vi "Set 2D Ramp Rates.vi"(0 "Y-Axis Communications Config":T1={"GPIB address"=22, "GPIB bus"=0, "connection ID"=refnum, "IP"="192.168.2.200", "Active Comm Interface"=0, "Serial Port"="", "Programmer Type"=0} {"Programmer Type" items=["Model 430", "Model 420"]; "Active Comm Interface" items=["TCP/IP (Model 430 Only)", "RS232", "IEEE488"]}, 1 "Y-Axis Field (kG)":dbl format="%.3f", 3 "Next Y-Axis Field (kG)":dbl format="%.3f", 4 "Z-Axis Communications Config":T1={"GPIB address"=22, "GPIB bus"=0, "connection ID"=refnum, "IP"="192.168.2.200", "Active Comm Interface"=0, "Serial Port"="", "Programmer Type"=0} {"Programmer Type" items=["Model 430", "Model 420"]; "Active Comm Interface" items=["TCP/IP (Model 430 Only)", "RS232", "IEEE488"]}, 5 "Z-Axis Field (kG)":dbl format="%.3f", 7 "Next Z-Axis Field (kG)":dbl format="%.3f", 8 "Max Ramp Rate - Y Axis (A/s)":dbl format="%.3f", 9 "Max Ramp Rate - Z Axis (A/s)":dbl format="%.3f", 11 "error in":T2) -> (15 "Y-Axis Ramp Rate (kG/s)":dbl format="%.3f", 17 "Z-Axis Ramp Rate (kG/s)":dbl format="%.3f", 18 "error out":T2)   [LabVIEW 2016]
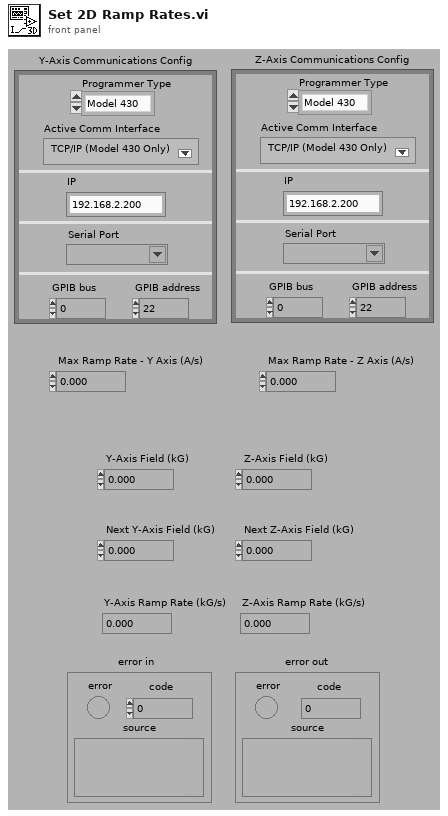
[diagram p1: front panel]
types:
  T1 = cluster{"GPIB address":i16, "GPIB bus":i16, "connection ID":refnum<k5>, "IP":string, "Active Comm Interface":u16, "Serial Port":refnum<visa-resource-name>, "Programmer Type":u16}
  T2 = cluster{"error":bool, "code":i32, "source":string}
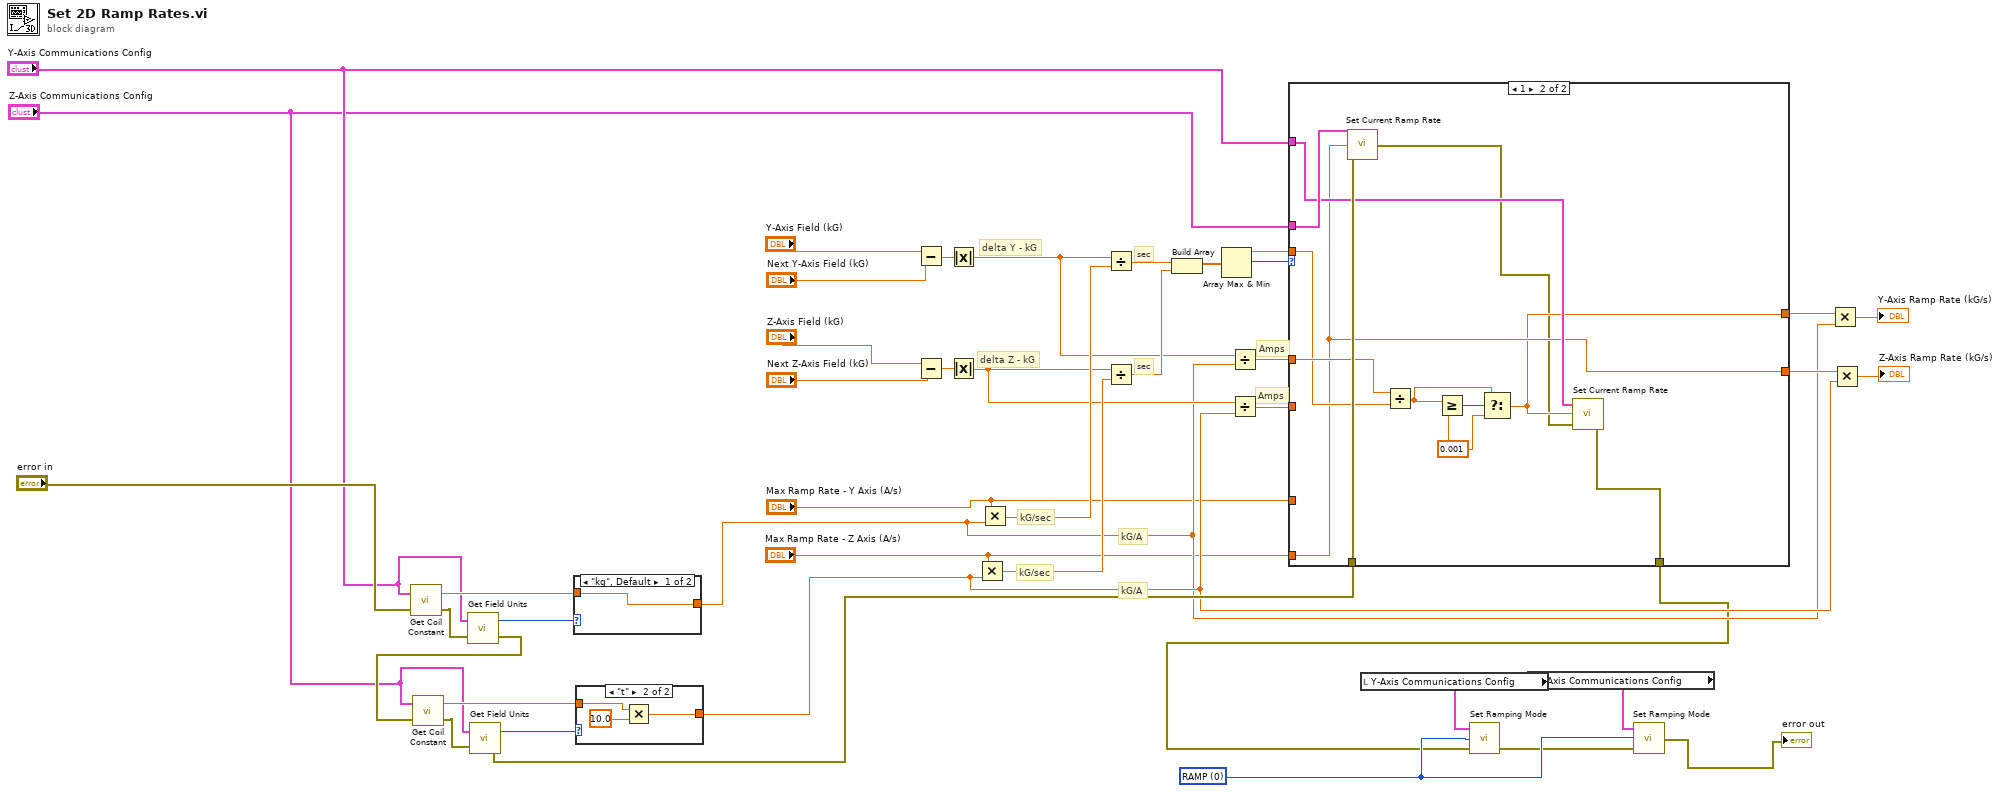
[diagram p0: block diagram]
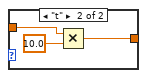
[diagram p3: hidden frame]
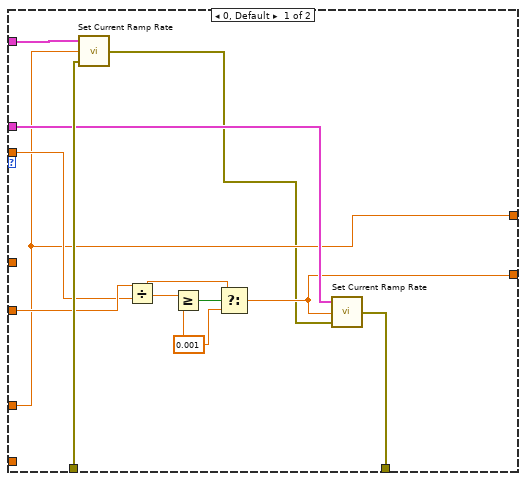
[diagram p4: hidden frame]
diagram:
  w21 = u16 0 items=["RAMP", "PAUSE", "MANUAL UP", "MANUAL DOWN", "ZERO"] ("Ramping Mode")
  # "kG/A"
  # "kG/A"
  # "kG/sec"
  # "kG/sec"
  # "Amps"
  # "Amps"
  # "delta Z - kG"
  # "delta Y - kG"
  # "sec"
  # "sec"
  n1 = call "Get Coil Constant.vi"("error in"="error in", "Communications Config"="Y-Axis Communications Config") -> ("error out"=w14:T2, "Coil Constant"=w15:dbl)
  n2 = call "Get Field Units.vi"("error in"=w14, "Z-Axis Communications Config"="Y-Axis Communications Config") -> ("error out"=w10:T2, "Field Units"=w16:enum16{"kg", "t"})
  n3 = call "Get Coil Constant.vi"("error in"=w10, "Communications Config"="Z-Axis Communications Config") -> ("error out"=w11:T2, "Coil Constant"=w12:dbl)
  n4 = call "Get Field Units.vi"("error in"=w11, "Z-Axis Communications Config"="Z-Axis Communications Config") -> ("error out"=w9:T2, "Field Units"=w13:enum16{"kg", "t"})
  n5 = case shown="\"kg\", Default" w16 {
    tunnel: w15 -> [w43 w45]
    tunnel: [w43 w44] -> w7
    frame "kg", Default {
    }
    frame "t" {
      n6 = Multiply(x=w45, y=10.0) -> (x*y=w44:dbl)
    }
  }
  n7 = case shown="\"t\"" w13 {
    tunnel: w12 -> [w47 w49]
    tunnel: [w47 w48] -> w8
    frame "kg", Default {
    }
    frame "t" {
      n8 = Multiply(x=w49, y=10.0) -> (x*y=w48:dbl)
    }
  }
  n9 = Subtract(x="Y-Axis Field (kG)", y="Next Y-Axis Field (kG)") -> (x-y=w33:dbl)
  n10 = Subtract(x="Z-Axis Field (kG)", y="Next Z-Axis Field (kG)") -> (x-y=w32:dbl)
  n11 = Absolute Value(x=w33) -> (abs(x)=w30:dbl)
  n12 = Absolute Value(x=w32) -> (abs(x)=w29:dbl)
  n13 = Multiply(x="Max Ramp Rate - Z Axis (A/s)", y=w8) -> (x*y=w41:dbl)
  n14 = Multiply(x="Max Ramp Rate - Y Axis (A/s)", y=w7) -> (x*y=w42:dbl)
  n15 = Divide(x=w30, y=w42) -> (x/y=w40:dbl)
  n16 = Divide(x=w29, y=w41) -> (x/y=w39:dbl)
  n17 = Build Array(w40, w39) -> (w31:dbl[])
  n18 = Array Max & Min(array=w31) -> (max value=w28:dbl, max index (indices)=w34:i32)  [unwired: 2 out]
  n19 = Divide(x=w30, y=w7) -> (x/y=w27:dbl)
  n20 = Divide(x=w29, y=w8) -> (x/y=w26:dbl)
  n21 = case shown="1" w34 {
    tunnel: w9 -> [w61 w73]
    tunnel: w28 -> [w59 w71]
    tunnel: w27 -> [_ w72]
    tunnel: "Y-Axis Communications Config" -> [w62 w70]
    tunnel: w26 -> [w60 _]
    tunnel: "Z-Axis Communications Config" -> [w58 w74]
    tunnel: [w57 w69] -> w3
    tunnel: [w56 w64] -> w25
    tunnel: [w52 w68] -> w24
    tunnel: "Max Ramp Rate - Y Axis (A/s)" -> [w56 _]
    tunnel: "Max Ramp Rate - Z Axis (A/s)" -> [_ w68]
    frame 0, Default {
      w55 = 0.001 ("f")
      n22 = call "Set Current Ramp Rate.vi"("Communications Config"=w62, "Ramp Rate (A/sec)"=w56, "error in"=w61) -> ("error out"=w51:T2)  [unwired: 2 in]
      n23 = Divide(x=w60, y=w59) -> (x/y=w53:dbl)
      n24 = Greater Or Equal?(x=w53, y=w55) -> (x >= y?=w54:bool)
      n25 = Select(t=w53, s=w54, f=w55) -> (s? t:f=w52:dbl)
      n26 = call "Set Current Ramp Rate.vi"("Communications Config"=w58, "Ramp Rate (A/sec)"=w52, "error in"=w51) -> ("error out"=w57:T2)  [unwired: 2 in]
    }
    frame 1 {
      w67 = 0.001 ("f")
      n27 = call "Set Current Ramp Rate.vi"("Communications Config"=w74, "Ramp Rate (A/sec)"=w68, "error in"=w73) -> ("error out"=w63:T2)  [unwired: 2 in]
      n28 = Divide(x=w72, y=w71) -> (x/y=w65:dbl)
      n29 = Greater Or Equal?(x=w65, y=w67) -> (x >= y?=w66:bool)
      n30 = Select(t=w65, s=w66, f=w67) -> (s? t:f=w64:dbl)
      n31 = call "Set Current Ramp Rate.vi"("Communications Config"=w70, "Ramp Rate (A/sec)"=w64, "error in"=w63) -> ("error out"=w69:T2)  [unwired: 2 in]
    }
  }
  n32 = local read "Y-Axis Communications Config"() -> (w19:T1)
  n33 = call "Set Ramping Mode.vi"("error in"=w3, "Ramping Mode"=w21, "Communications Config"=w19) -> ("error out"=w20:T2)
  n34 = local read "Z-Axis Communications Config"() -> (w18:T1)
  n35 = call "Set Ramping Mode.vi"("error in"=w20, "Ramping Mode"=w21, "Communications Config"=w18) -> ("error out"=→"error out":T2)
  n36 = Multiply(x=w25, y=w7) -> (x*y=→"Y-Axis Ramp Rate (kG/s)":dbl)
  n37 = Multiply(x=w24, y=w8) -> (x*y=→"Z-Axis Ramp Rate (kG/s)":dbl)
